vi "deadbanding.vi"(10 "width":dbl, 11 "joystick":dbl) -> (3 "deadbanded":dbl)   [LabVIEW 2014]
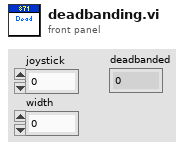
[diagram p1: front panel]
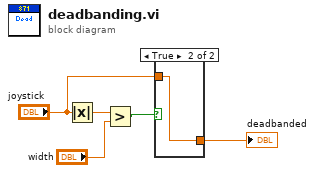
[diagram p0: block diagram]
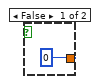
[diagram p2: hidden frame]
diagram:
  n1 = Absolute Value(x="joystick") -> (abs(x)=w4:dbl)
  n2 = Greater?(x=w4, y="width") -> (0:w2:bool)
  n3 = case shown="True" w2 {
    tunnel: [0 w7] -> w5
    tunnel: "joystick" -> [_ w7]
    frame False {
    }
    frame True {
    }
  }
  "deadbanded" <- w5
